vi "Create Grid.vi"(10 "input cluster":T1) -> (3 "Grid out":refnum<class "Grid.lvclass">)   [LabVIEW 2016, in "Grid.lvclass"]
uses:
  Grid.lvclass
  Pixel/Pixel.lvclass
panel:
  out "Pixels Remaining":i32
  out "Loops Remaining":i32
  out "size(s)":i32[](array[numeric])
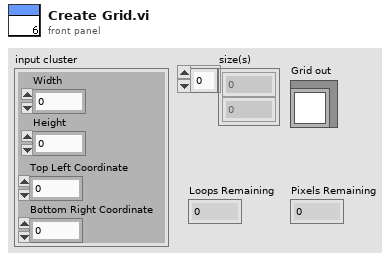
[diagram p1: front panel]
types:
  T1 = cluster{"Width":i32, "Height":i32, "Top Left Coordinate":cdb, "Bottom Right Coordinate":cdb}
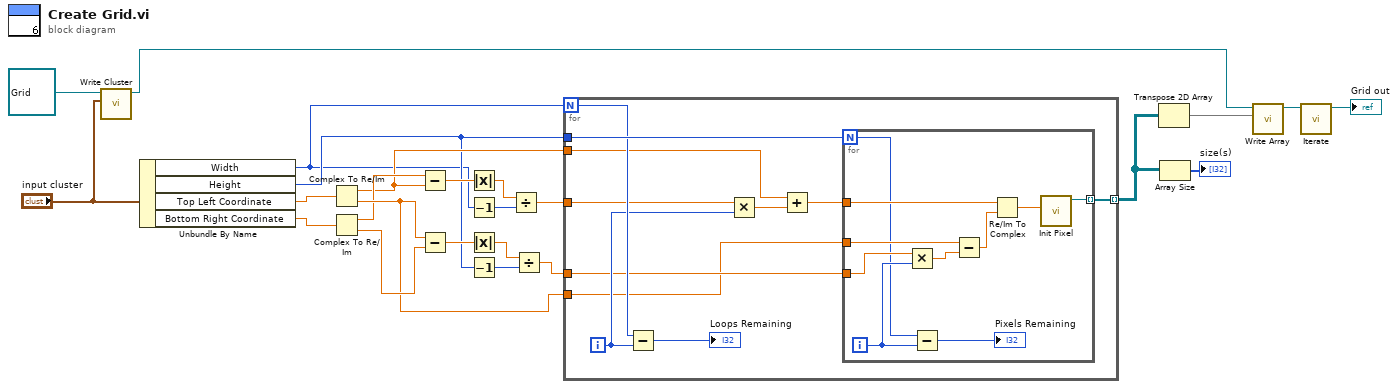
[diagram p0: block diagram]
diagram:
  n1 = call-dynamic "Write Cluster.vi"("Grid Parameters"="input cluster", "Grid in"=refnum<class "Grid.lvclass"> refnum) -> ("Grid out"=w2:refnum<class "Grid.lvclass">)  [unwired: 8 in, 1 out]
  n2 = Unbundle By Name("input cluster") -> ("Width"=w7:i32, "Height"=w8:i32, "Top Left Coordinate"=w10:cdb, "Bottom Right Coordinate"=w9:cdb)
  n3 = Complex To Re/Im(x + iy=w10) -> (x=w11:dbl, y=w13:dbl)
  n4 = Complex To Re/Im(x + iy=w9) -> (x=w12:dbl, y=w14:dbl)
  n5 = Subtract(x=w12, y=w11) -> (x-y=w16:dbl)
  n6 = Subtract(x=w13, y=w14) -> (x-y=w22:dbl)
  n7 = Absolute Value(x=w16) -> (abs(x)=w17:dbl)
  n8 = Decrement(x=w7) -> (x-1=w18:i32)
  n9 = Absolute Value(x=w22) -> (abs(x)=w21:dbl)
  n10 = Decrement(x=w8) -> (x-1=w19:i32)
  n11 = Divide(x=w17, y=w18) -> (x/y=w15:dbl)
  n12 = Divide(x=w21, y=w19) -> (x/y=w20:dbl)
  n13 = for {
    N: w7 -> [w32]
    tunnel: [w35] -> w23 mode=indexing
    tunnel: w8 -> [w34]
    tunnel: w20 -> [w26]
    tunnel: w15 -> [w30]
    tunnel: w11 -> [w31]
    tunnel: w13 -> [w25]
    i -> [w29]
    n14 = Subtract(x=w32, y=w29) -> (x-y=→"Loops Remaining":i32)
    n15 = Multiply(x=w30, y=w29) -> (x*y=w28:dbl)
    n16 = Add(x=w31, y=w28) -> (x+y=w27:dbl)
    n17 = for {
      N: w34 -> [w36]
      tunnel: [w45] -> w35 mode=indexing
      tunnel: w27 -> [w43]
      tunnel: w26 -> [w41]
      tunnel: w25 -> [w40]
      i -> [w37]
      n18 = Multiply(x=w41, y=w37) -> (x*y=w42:dbl)
      n19 = Subtract(x=w36, y=w37) -> (x-y=→"Pixels Remaining":i32)
      n20 = Subtract(x=w40, y=w42) -> (x-y=w39:dbl)
      n21 = Re/Im To Complex(1:w39, 2:w43) -> (0:w44:cdb)
      n22 = call "Init Pixel.vi"("Coordinate"=w44) -> ("Pixel"=w45:refnum<class "Pixel.lvclass">)  [unwired: 10 in]
    }
  }
  n23 = Transpose 2D Array(2D array=w23) -> (transposed array=w6:refnum<class "Pixel.lvclass">[][])
  n24 = Array Size(array=w23) -> (size(s)=→"size(s)":i32[])
  n25 = call-dynamic "Write Array.vi"("Grid"=w6, "Grid in"=w2) -> ("Grid out"=w5:refnum<class "Grid.lvclass">)  [unwired: 8 in, 1 out]
  n26 = call "Iterate.vi"("Grid.lvclass 2"=w5) -> ("Grid.lvclass"=→"Grid out":refnum<class "Grid.lvclass">)  [unwired: 10 in]
